vi "RT_Gravitational_Force_in_DLR_Body_Reference_System (SubVI).vi"(10 "DCM":dbl[][](array[numeric]), 11 "FG_d":dbl[](array[numeric])) -> (3 "FG_b":dbl[](array[numeric]))   [LabVIEW 2017]
uses:
  <vilib>/Analysis/baseanly.llb/Real A x B.vi
  <vilib>/Analysis/Matrix/Numeric/Conversions/Array To Matrix - RA.vi
  <vilib>/Analysis/Matrix/Numeric/Conversions/Array To Matrix - RA2.vi
  <vilib>/Analysis/Matrix/Numeric/Conversions/Matrix To Array - RM.vi
  <vilib>/Analysis/NI_AALBase.lvlib
  <vilib>/Analysis/Matrix/NI_Matrix.lvlib
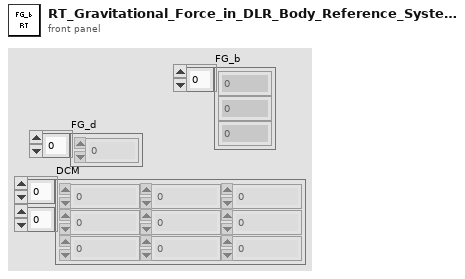
[diagram p1: front panel]
types:
  T1 = typedef "NI_Matrix.lvlib/RealMatrix.ctl" = dbl[][]
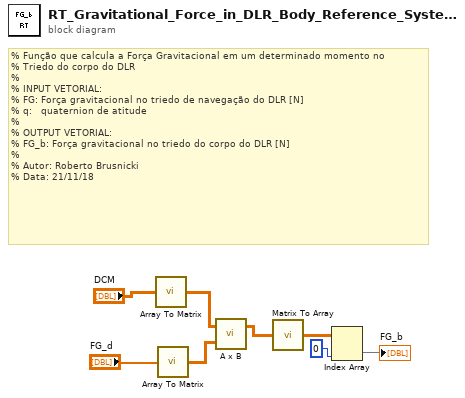
[diagram p0: block diagram]
diagram:
  # "% Função que calcula a Força Gravitacional em um determinado momento no \n% Triedo do corpo do DLR\n%\n% INPUT VETORIAL: \n% FG: Força gravitacional no triedo de navegação do DLR [N]\n% q:   quaternion de atitude   \n%\n% OUTPUT VETORIAL:\n% FG_b: Força gravitacional no triedo do corpo do DLR [N]\n%\n% Autor: Roberto Brusnicki\n% Data: 21/11/18"
  n1 = call-poly <vilib>:"Array To Matrix.vi"("Real 2D Array"="DCM") -> ("Real Matrix"=w6:T1)
  n2 = call-poly <vilib>:"Array To Matrix.vi"("Real 1D Array"="FG_d") -> ("Real Matrix (Column Vector)"=w3:T1)
  n3 = call-poly <vilib>:"A x B.vi"("B"=w3, "A"=w6) -> ("A x B"=w8:T1)  [unwired: 1 out]
  n4 = call-poly <vilib>:"Matrix To Array.vi"("Real Matrix"=w8) -> ("Real 2D Array"=w4:dbl[][])
  n5 = Index Array(array=w4, index (col)=0 ("index (row)")) -> (element=→"FG_b":dbl[])  [unwired: 1 in]
